vi "Generate Output.vi"(2 "Input":dbl, 3 "PIDClass.lvclass":refnum<class "PIDClass.lvclass">) -> (0 "Output":dbl, 1 "PIDClass.lvclass out":refnum<class "PIDClass.lvclass">)   [LabVIEW 2011, in "PIDClass.lvclass"]
uses:
  PIDClass.lvclass
  PIDClass.lvclass/PIDClass.ctl
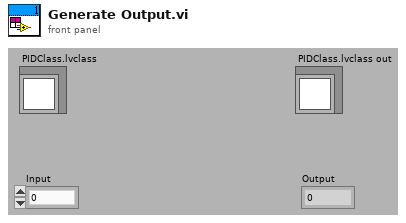
[diagram p1: front panel]
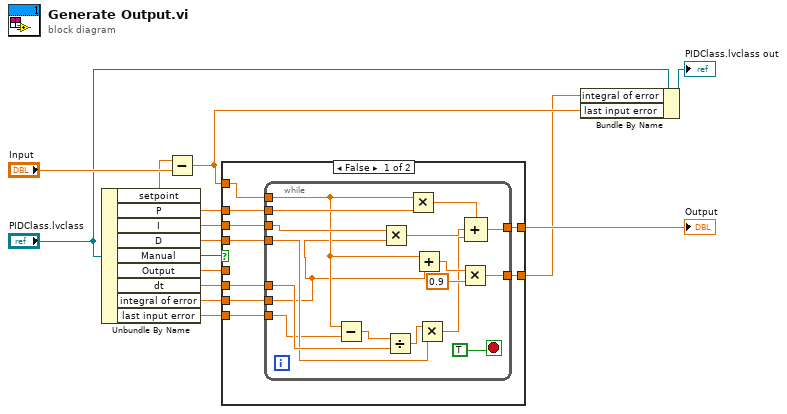
[diagram p0: block diagram]
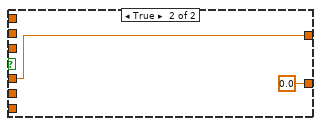
[diagram p2: hidden frame]
diagram:
  n1 = Unbundle By Name("PIDClass.lvclass") -> ("setpoint"=w7:dbl, "P"=w12:dbl, "I"=w11:dbl, "D"=w10:dbl, "Manual"=w15:bool, "Output"=w14:dbl, "dt"=w9:dbl, "integral of error"=w2:dbl, "last input error"=w3:dbl)
  n2 = Subtract(x=w7, y="Input") -> (x-y=w4:dbl)
  n3 = case shown="False" w15 {
    tunnel: w14 -> [_ w43]
    tunnel: [w24 w43] -> w13
    tunnel: w12 -> [w23 _]
    tunnel: w11 -> [w21 _]
    tunnel: w10 -> [w19 _]
    tunnel: w4 -> [w22 _]
    tunnel: w9 -> [w20 _]
    tunnel: w3 -> [w18 _]
    tunnel: w2 -> [w17 _]
    tunnel: [w16 0.0] -> w1
    frame False {
      n4 = while {
        tunnel: [w41] -> w24
        tunnel: w23 -> [w40]
        tunnel: w22 -> [w27]
        tunnel: w21 -> [w35]
        tunnel: w20 -> [w32]
        tunnel: w19 -> [w30]
        tunnel: w18 -> [w28]
        tunnel: w17 -> [w26]
        tunnel: [w25] -> w16
        stop <- TRUE stop-if-true
        n5 = Subtract(x=w27, y=w28) -> (x-y=w33:dbl)
        n6 = Multiply(x=w35, y=w26) -> (x*y=w34:dbl)
        n7 = Divide(x=w33, y=w32) -> (x/y=w31:dbl)
        n8 = Multiply(x=w27, y=w40) -> (x*y=w39:dbl)
        n9 = Add(x=w27, y=w26) -> (x+y=w37:dbl)
        n10 = Multiply(x=w31, y=w30) -> (x*y=w29:dbl)
        n11 = Multiply(x=w37, y=0.9) -> (x*y=w25:dbl)
        n12 = Compound Arithmetic op=unknown(w39, w34, w29) -> (w41:dbl)
      }
    }
    frame True {
    }
  }
  "Output" <- w13
  n13 = Bundle By Name(cluster="PIDClass.lvclass", "integral of error"=w1, "last input error"=w4) -> (→"PIDClass.lvclass out":refnum<class "PIDClass.lvclass">)
